vi "Replace Error.vi"(7 "scope":T3=enum."global", 8 "error in (no error)":errorcluster, 9 "new error":T2, 10 "error owner and ID":T1, 11 "error list <top> in":variant) -> (0 "error out":errorcluster, 3 "error list <top> out":variant)   [LabVIEW 2017]
uses:
  Scope.ctl
  Error File Management/Controls/NI Error.ctl
  Error Owner and ID.ctl
  Error File Management/Error File Management.lvlib
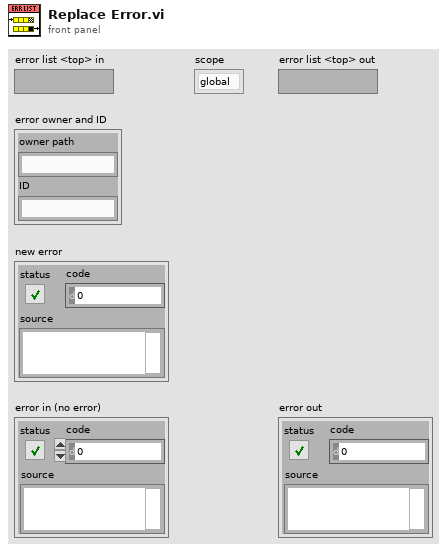
[diagram p1: front panel]
types:
  T1 = typedef "Error Owner and ID.ctl" = cluster{"owner path":string, "ID":string}
  T2 = typedef "Error File Management.lvlib/NI Error.ctl" = errorcluster
  T3 = typedef "Scope.ctl" = enum16{"project", "global"}
  T4 = typedef "Error Code File Properties.ctl" = cluster{"path":path, "simplified path":string, "name":string, "display name":string, "family name":string, "comment":string, "parsable?":bool, "file modified?":bool}
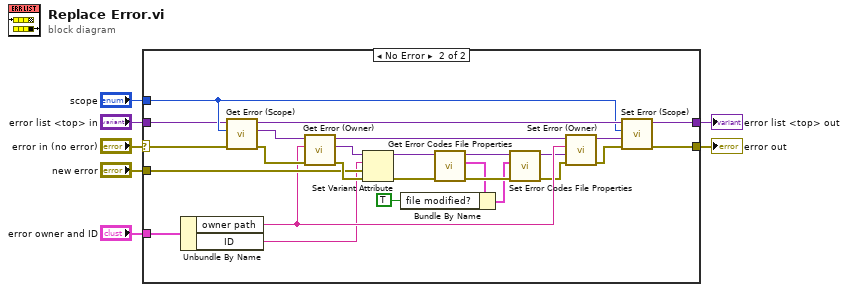
[diagram p0: block diagram]
diagram:
  n1 = case shown="No Error" "error in (no error)" {
    selector: "error in (no error)" -> [w9 w29]
    tunnel: "scope" -> [_ w31]
    tunnel: [w9 w30] -> w5
    tunnel: "error list <top> in" -> [w8 w28]
    tunnel: [w8 w27] -> w3
    tunnel: "new error" -> [_ w23]
    tunnel: "error owner and ID" -> [_ w22]
    frame Error {
    }
    frame No Error {
      n2 = Unbundle By Name(w22) -> ("owner path"=w21:string, "ID"=w20:string)
      n3 = call "Get Error (Scope).vi"("error in (no error)"=w29, "scope"=w31, "error list <top>"=w28) -> ("error out"=w32:errorcluster, "error list <scope>"=w34:variant, "error list <top> dup"=w33:variant)  [unwired: 5 in, 1 out]
      n4 = call "Get Error (Owner).vi"("error in (no error)"=w32, "owner"=w21, "error list <scope>"=w34) -> ("error out"=w24:errorcluster, "error list <owner>"=w25:variant, "error list <scope> dup"=w26:variant)  [unwired: 5 in, 1 out]
      n5 = Set Variant Attribute(Variant=w25, name=w20, value=w23, error in=w24) -> (Variant out=w14:variant, error out=w13:errorcluster)  [unwired: 1 out]
      n6 = call "Get Error Codes File Properties.vi"("error in (no error)"=w13, "error list <owner> in"=w14) -> ("error out"=w35:errorcluster, "properties"=w16:T4, "error list <owner> out"=w17:variant)  [unwired: 6 in, 1 out]
      n7 = Bundle By Name(cluster=w16, "file modified?"=TRUE) -> (w18:T4)
      n8 = call "Set Error Codes File Properties.vi"("error in (no error)"=w35, "properties"=w18, "error list <owner> in"=w17) -> ("error out"=w11:errorcluster, "error list <owner> out"=w12:variant)  [unwired: 7 in]
      n9 = call "Set Error (Owner).vi"("error in (no error)"=w11, "error list <owner>"=w12, "owner"=w21, "error list <scope> in"=w26) -> ("error out"=w10:errorcluster, "error list <scope> out"=w15:variant)  [unwired: 6 in]
      n10 = call "Set Error (Scope).vi"("error in (no error)"=w10, "error list <scope>"=w15, "scope"=w31, "error list <top> in"=w33) -> ("error out"=w30:errorcluster, "error list <top> out"=w27:variant)  [unwired: 6 in]
    }
  }
  "error out" <- w5
  "error list <top> out" <- w3
